vi "Coppia da potenza.vi"(10 "Pmecc W":dbl, 11 "RPM letti":dbl) -> (3 "t":dbl)   [LabVIEW 2019]
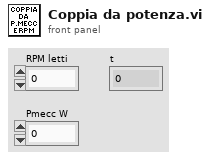
[diagram p1: front panel]
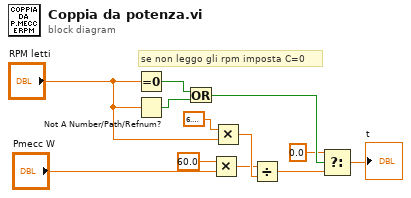
[diagram p0: block diagram]
diagram:
  # "se non leggo gli rpm imposta C=0"
  n1 = Equal To 0?(x="RPM letti") -> (x = 0?=w4:bool)
  n2 = Not A Number/Path/Refnum?(number/path/refnum="RPM letti") -> (NaN/Path/Refnum?=w10:bool)
  n3 = Or(x=w4, y=w10) -> (x .or. y?=w11:bool)
  n4 = Multiply(x=60.0, y="Pmecc W") -> (x*y=w5:dbl)
  n5 = Multiply(x=6.283185307179586, y="RPM letti") -> (x*y=w6:dbl)
  n6 = Divide(x=w5, y=w6) -> (x/y=w3:dbl)
  n7 = Select(t=0.0, s=w11, f=w3) -> (s? t:f=→"t":dbl)
